vi "Create Arbitrary Waveform [ARB].vi"(8 "error in (no error)":errorcluster, 9 "waveform data array (empty)":dbl[](array[numeric]) format="%.3f", 11 "CS++Fgen in":refnum<class "CS++Fgen.lvclass">) -> (0 "error out":errorcluster, 2 "waveform handle":i32, 3 "CS++Fgen out":refnum<class "CS++Fgen.lvclass">)   [LabVIEW 2016, in "CS++Fgen.lvlib" / "CS++Fgen.lvclass"]
doc: "This VI creates an arbitrary waveform and returns a handle that identifies that waveform. You pass this handle to the IviFgen Configure Arbitrary Waveform [ARB] VI to produce that waveform. You also use the handles this VI returns to specify a sequence of arbitrary waveforms with the IviFgen Create Arbitrary Sequence [SEQ] VI.\n\nNotes:\n\n(1) This VI is part of the IviFgenArbWfm [ARB] extension group."
uses:
  CS++Fgen.lvclass
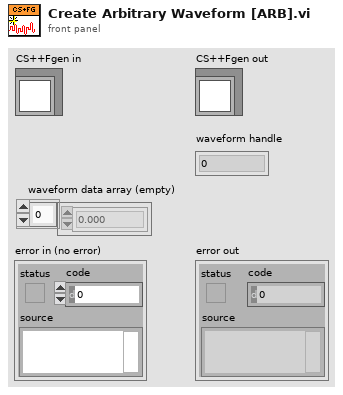
[diagram p1: front panel]
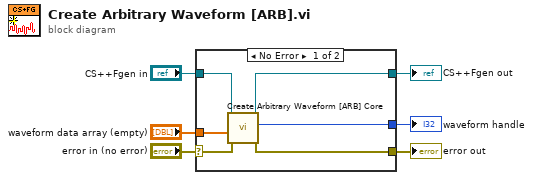
[diagram p0: block diagram]
diagram:
  n1 = case shown="No Error" "error in (no error)" {
    selector: "error in (no error)" -> [w10 w14]
    tunnel: [w9 w14] -> w5
    tunnel: [w11 w13] -> w3
    tunnel: "CS++Fgen in" -> [w12 w13]
    tunnel: "waveform data array (empty)" -> [w8 _]
    tunnel: [w7 _] -> w1
    frame No Error {
      n2 = call-dynamic "Create Arbitrary Waveform [ARB] Core.vi"("error in (no error)"=w10, "waveform data array (empty)"=w8, "CS++Fgen in"=w12) -> ("error out"=w9:errorcluster, "waveform handle"=w7:i32, "CS++Fgen out"=w11:refnum<class "CS++Fgen.lvclass">)  [unwired: 6 in]
    }
    frame Error {
    }
  }
  "error out" <- w5
  "CS++Fgen out" <- w3
  "waveform handle" <- w1
